vi "Smart Umbrella.vi"() -> ()   [LabVIEW 2022 SP3]
uses:
  <vilib>/DAQmx/read.llb/DAQmx Read (Digital Bool 1Line 1Point).vi
  <vilib>/DAQmx/write.llb/DAQmx Write (Digital Bool 1Line 1Point).vi
  <vilib>/DAQmx/read.llb/DAQmx Read (Analog 1D DBL NChan 1Samp).vi
  <vilib>/DAQmx/create/channels.llb/DAQmx Create Channel (AI-Voltage-Basic).vi
  <vilib>/DAQmx/miscellaneous.llb/DAQmx Fill In Error Info.vi
  <vilib>/DAQmx/create/channels.llb/DAQmx Create Channel (DO-Digital Output).vi
  <vilib>/DAQmx/create/channels.llb/DAQmx Create Channel (DI-Digital Input).vi
panel:
  out "Pressure":dbl(knob) scale=0.0..5.0
  out "Voltage Output of AMT1001":dbl(knob) scale=0.0..5.0
  out "Bag Status\nWorn/Not":bool
  in  "stop 3":bool
  out "Button h":bool
  in  "Button":tag
  in  "stop 2":bool
  in  "stop (F)":bool
  out "Square":dynamicdata(graph)
  in  "Frequency":dbl=50.0
  in  "Offset":dbl=2.5
  in  "Amplitude":dbl=2.5
  out "Buzzer Light":bool
  out "x .and. y? 6":bool
  in  "Buzzer":tag
  out "Fold/Unfold":bool
  out "Rain Status Indicator":bool
  out "Humidity Level Indicator":bool
  out "Rain Sensor Voltage Output":dbl(knob) scale=0.0..5.0
  out "Humidity Level":dbl(knob) scale=0.0..100.0
  in  "stop":bool
  in  "Analog Pins":tag
  # "SMART UMBRELLA"
  # "Rain Status"
  # "Humidity"
  # "Bag Wearing Detection"
  # "Umbrella Position Indicator"
  # "Configuration"
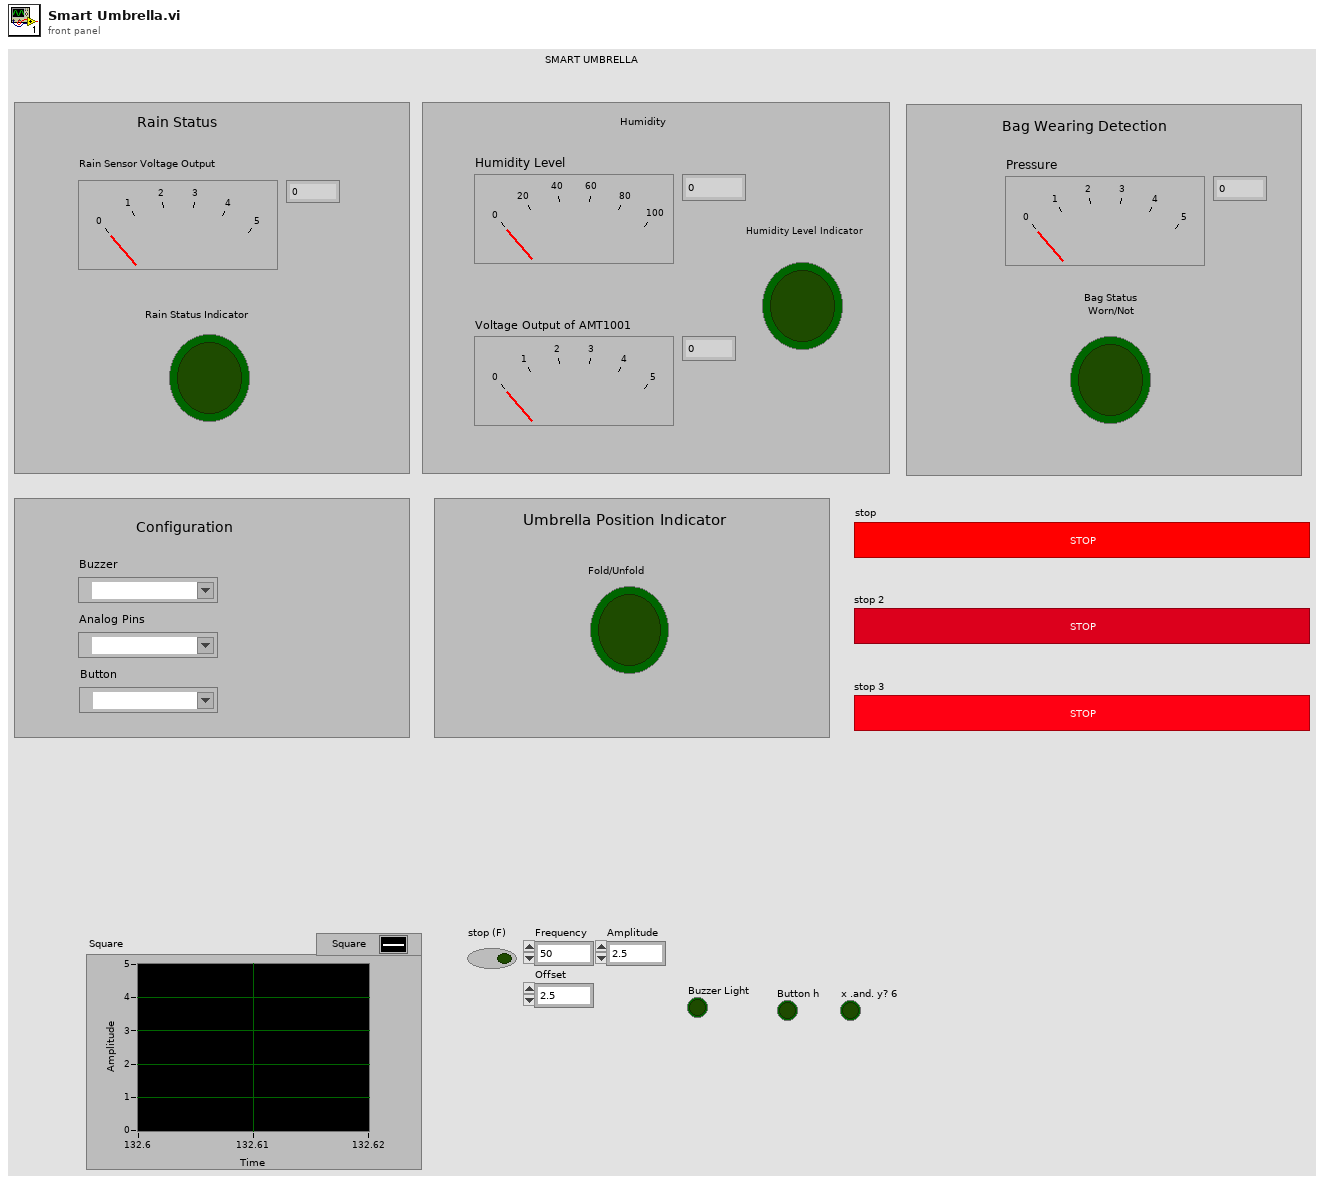
[diagram p1: front panel]
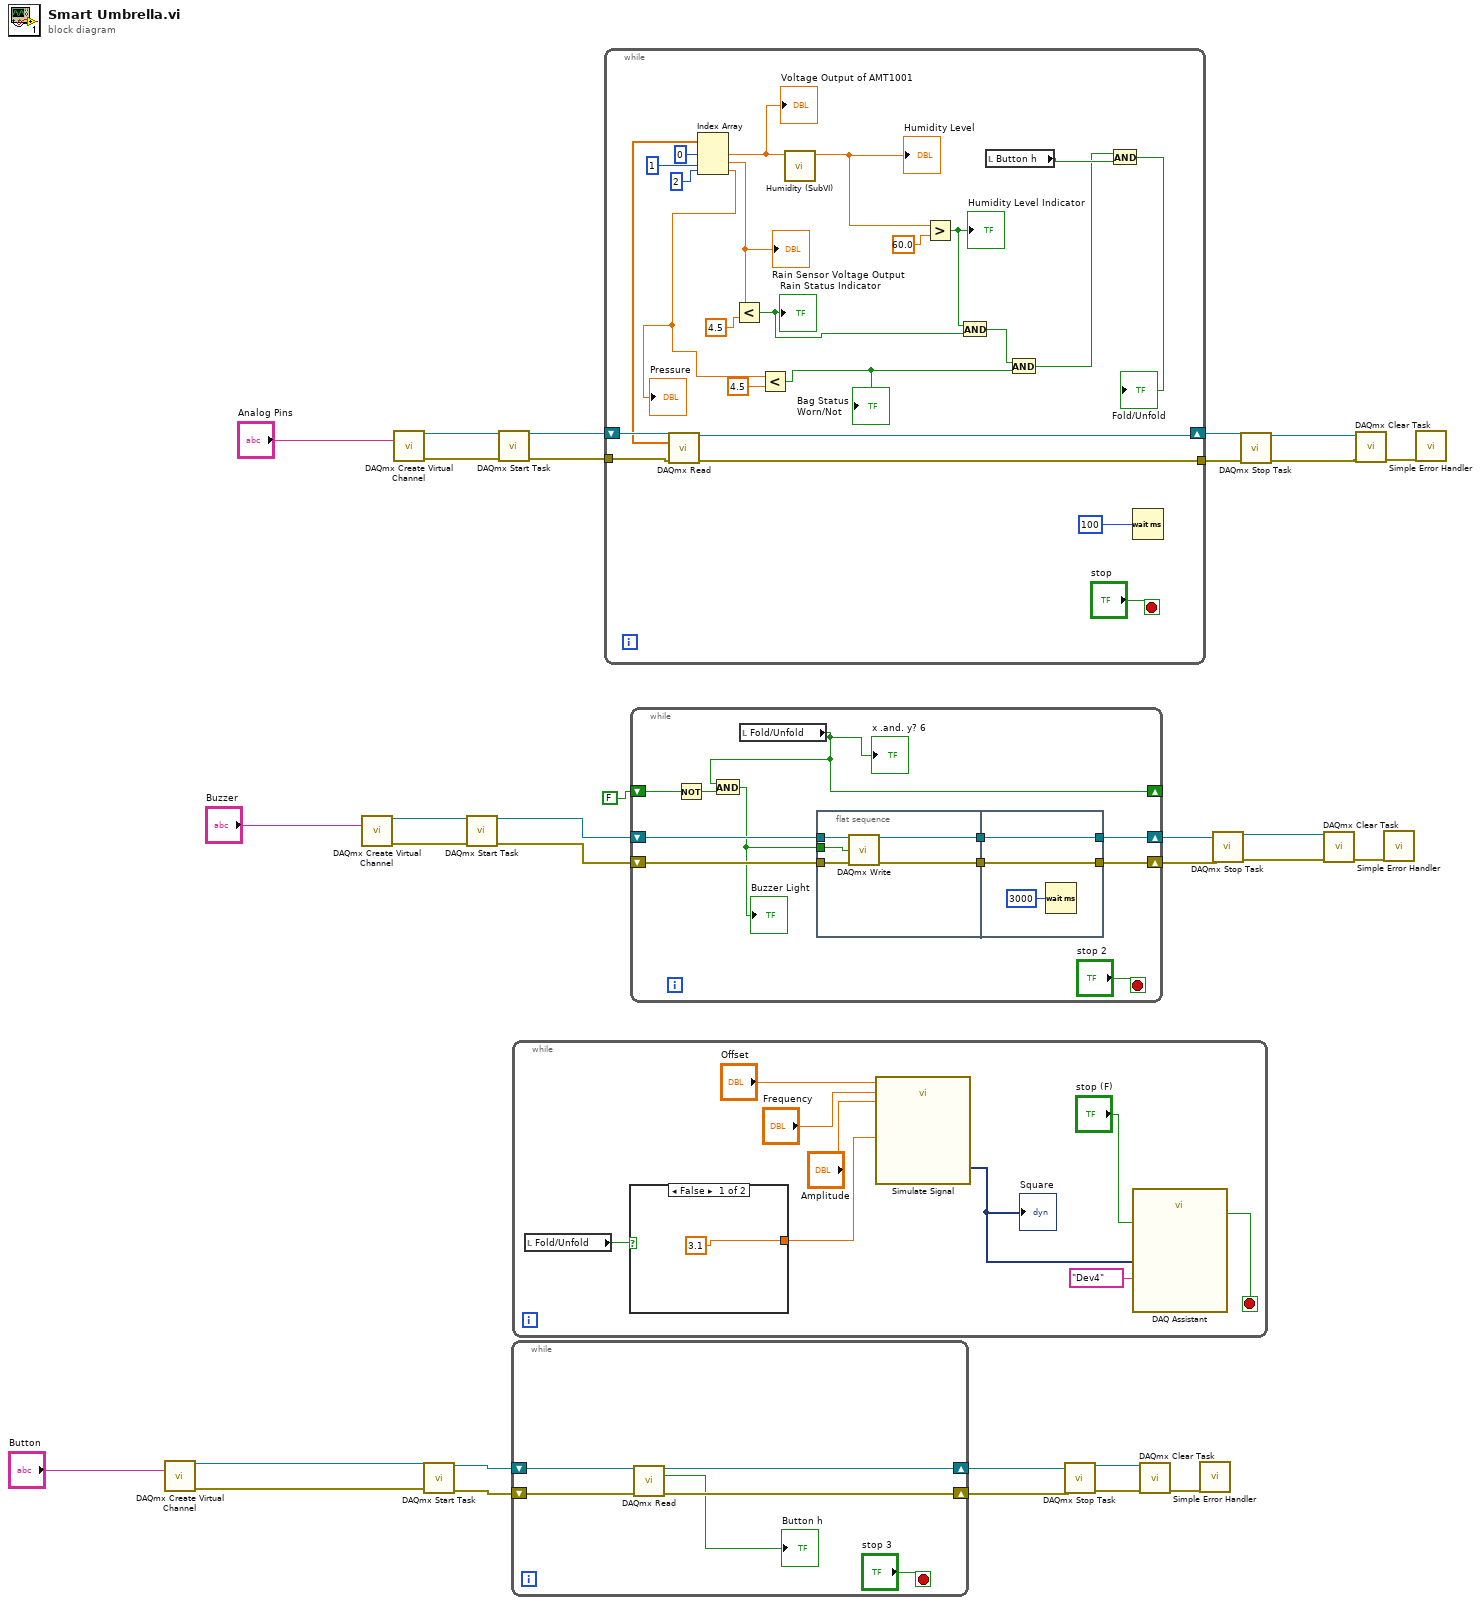
[diagram p0: block diagram]
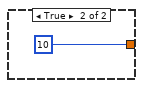
[diagram p2: hidden frame]
diagram:
  n1 = call-poly <vilib>:"DAQmx Create Virtual Channel.vi"("lines"="Button") -> ("task out"=w2:refnum<k21>, "error out"=w1:errorcluster)  [unwired: 13 in]
  n2 = call-poly <vilib>:"DAQmx Create Virtual Channel.vi"("lines"="Buzzer") -> ("task out"=w20:refnum<k21>, "error out"=w19:errorcluster)  [unwired: 13 in]
  n3 = call-poly <vilib>:"DAQmx Create Virtual Channel.vi"("physical channels"="Analog Pins") -> ("task out"=w30:refnum<k21>, "error out"=w27:errorcluster)  [unwired: 13 in]
  n4 = call <vilib>:"DAQmx Start Task.vi"("task/channels in"=w2, "error in"=w1) -> ("task out"=w6:refnum<k21>, "error out"=w5:errorcluster)  [unwired: 12 in]
  n5 = call <vilib>:"DAQmx Start Task.vi"("task/channels in"=w20, "error in"=w19) -> ("task out"=w15:refnum<k21>, "error out"=w14:errorcluster)  [unwired: 12 in]
  n6 = call <vilib>:"DAQmx Start Task.vi"("task/channels in"=w30, "error in"=w27) -> ("task out"=w29:refnum<k21>, "error out"=w26:errorcluster)  [unwired: 12 in]
  n7 = while {
    shift-right: [w35] -> w4
    shift-left: w6 -> [w37]
    shift-right: [w34] -> w3
    shift-left: w5 -> [w36]
    stop <- "stop 3" stop-if-true
    n8 = call-poly <vilib>:"DAQmx Read.vi"("task/channels in"=w37, "error in"=w36) -> ("task out"=w35:refnum<k21>, "data"=→"Button h":bool, "error out"=w34:errorcluster)  [unwired: 11 in]
  }
  n9 = while {
    stop <- w45 stop-if-true
    n10 = local read "Fold/Unfold"() -> (w38:bool)
    n11 = case shown="False" w38 {
      tunnel: [3.1 10] -> w39
      frame False {
      }
      frame True {
      }
    }
    n12 = call "Simulate Signal"("Offset"="Offset", "Duty Cycle (%)"=w39, "Frequency"="Frequency", "Amplitude"="Amplitude") -> ("Square"=w41:dynamicdata)  [unwired: 10 in, 1 out]
    "Square" <- w41
    n13 = call "DAQ Assistant"("data"=w41, "stop (F)"="stop (F)", "device name"=tag "Dev4") -> ("stopped"=w45:bool)  [unwired: 14 in, 2 out]
  }
  n14 = while {
    shift-right: [w70] -> w28
    shift-left: w29 -> [w71]
    tunnel: w26 -> [w69]
    tunnel: [w68] -> w25
    stop <- "stop" stop-if-true
    n15 = call-poly <vilib>:"DAQmx Read.vi"("task/channels in"=w71, "error in"=w69) -> ("task out"=w70:refnum<k21>, "data"=w64:dbl[], "error out"=w68:errorcluster)  [unwired: 11 in]
    n16 = Index Array(array=w64, index #1=0 ("index"), index #2=1 ("index"), index #3=2 ("index")) -> (element #1=w50:dbl, element #2=w60:dbl, element #3=w49:dbl)
    "Rain Sensor Voltage Output" <- w60
    "Voltage Output of AMT1001" <- w50
    "Pressure" <- w49
    n17 = Less?(x=w60, y=4.5) -> (x < y?=w58:bool)
    "Rain Status Indicator" <- w58
    n18 = Less?(x=w49, y=4.5) -> (x < y?=w53:bool)
    "Bag Status\nWorn/Not" <- w53
    n19 = call "Humidity (SubVI).vi"("Waveform"=w50) -> ("Numeric"=w62:dbl)  [unwired: 10 in]
    "Humidity Level" <- w62
    n20 = Greater?(x=w62, y=60.0) -> (0:w59:bool)
    "Humidity Level Indicator" <- w59
    n21 = And(x=w59, y=w58) -> (x .and. y?=w51:bool)
    n22 = local read "Button h"() -> (w56:bool)
    n23 = And(x=w51, y=w53) -> (x .and. y?=w52:bool)
    n24 = And(x=w52, y=w56) -> (x .and. y?=→"Fold/Unfold":bool)
    n25 = Wait (ms)(milliseconds to wait=u32 100) -> ()  [unwired: 1 out]
  }
  n26 = while {
    shift-right: [w81] -> w13
    shift-left: w15 -> [w83]
    shift-right: [w80] -> w12
    shift-left: w14 -> [w82]
    shift-right: [w74] -> _
    shift-left: FALSE -> [w77]
    stop <- "stop 2" stop-if-true
    n27 = Not(x=w77) -> (.not. x?=w76:bool)
    n28 = local read "Fold/Unfold"() -> (w74:bool)
    "x .and. y? 6" <- w74
    n29 = And(x=w74, y=w76) -> (x .and. y?=w75:bool)
    "Buzzer Light" <- w75
    n30 = flat-sequence {
      tunnel: w83 -> [w88]
      tunnel: w82 -> [w87]
      tunnel: [w86] -> w79
      tunnel: [w85] -> w78
      tunnel: w75 -> [w84]
      tunnel: w79 -> [w91]
      tunnel: w78 -> [w90]
      tunnel: [w91] -> w81
      tunnel: [w90] -> w80
      frame #0 {
        n31 = call-poly <vilib>:"DAQmx Write.vi"("task/channels in"=w88, "data"=w84, "error in"=w87) -> ("task out"=w86:refnum<k21>, "error out"=w85:errorcluster)  [unwired: 10 in, 1 out]
      }
      frame #1 {
        n32 = Wait (ms)(milliseconds to wait=u32 3000) -> ()  [unwired: 1 out]
      }
    }
  }
  n33 = call <vilib>:"DAQmx Stop Task.vi"("task/channels in"=w4, "error in"=w3) -> ("task out"=w9:refnum<k21>, "error out"=w8:errorcluster)  [unwired: 12 in]
  n34 = call <vilib>:"DAQmx Clear Task.vi"("task in"=w9, "error in"=w8) -> ("error out"=w7:errorcluster)  [unwired: 13 in]
  n35 = call <vilib>:"Simple Error Handler.vi"("error in (no error)"=w7) -> ()  [unwired: 4 in, 5 out]
  n36 = call <vilib>:"DAQmx Stop Task.vi"("task/channels in"=w13, "error in"=w12) -> ("task out"=w18:refnum<k21>, "error out"=w17:errorcluster)  [unwired: 12 in]
  n37 = call <vilib>:"DAQmx Stop Task.vi"("task/channels in"=w28, "error in"=w25) -> ("task out"=w23:refnum<k21>, "error out"=w22:errorcluster)  [unwired: 12 in]
  n38 = call <vilib>:"DAQmx Clear Task.vi"("task in"=w18, "error in"=w17) -> ("error out"=w16:errorcluster)  [unwired: 13 in]
  n39 = call <vilib>:"DAQmx Clear Task.vi"("task in"=w23, "error in"=w22) -> ("error out"=w24:errorcluster)  [unwired: 13 in]
  n40 = call <vilib>:"Simple Error Handler.vi"("error in (no error)"=w16) -> ()  [unwired: 4 in, 5 out]
  n41 = call <vilib>:"Simple Error Handler.vi"("error in (no error)"=w24) -> ()  [unwired: 4 in, 5 out]
